vi "mono_camera_array1.vi"(0 "TCP Network Connection in":refnum<k5>, 1 "monoDrive Simulator IP":string, 2 "camera configurations input":T4={"Rear Camera"=path "C:/Users/celit/Documents/GitHub/client/configurations/camera/rear_camera.json", "Left Camera"=path "C:/Users/celit/Documents/GitHub/client/configurations/camera/left_camera.json", "Right Camera"=path "C:/Users/celit/Documents/GitHub/client/configurations/camera/right_camera.json", "Front Camera"=path "C:/Users/celit/Documents/GitHub/client/configurations/camera/front_camera.json", "Following Camera"=path "C:/Users/celit/Documents/GitHub/client/configurations/camera/follow_camera.json"}, 3 "error in (no error)":errorcluster) -> (4 "error out":errorcluster, 5 "camera responses output":T2, 6 "camera dimensions output":T1, 7 "camera connections output":T3, 8 "TCP Network Connection out":refnum<k5>)   [LabVIEW 2018, in "monoDrive.lvlib"]
uses:
  monoDrive.lvlib
panel:
  in  "camera dimensions define":T1
  in  "camera responses define":T2
  in  "camera connections define":T3
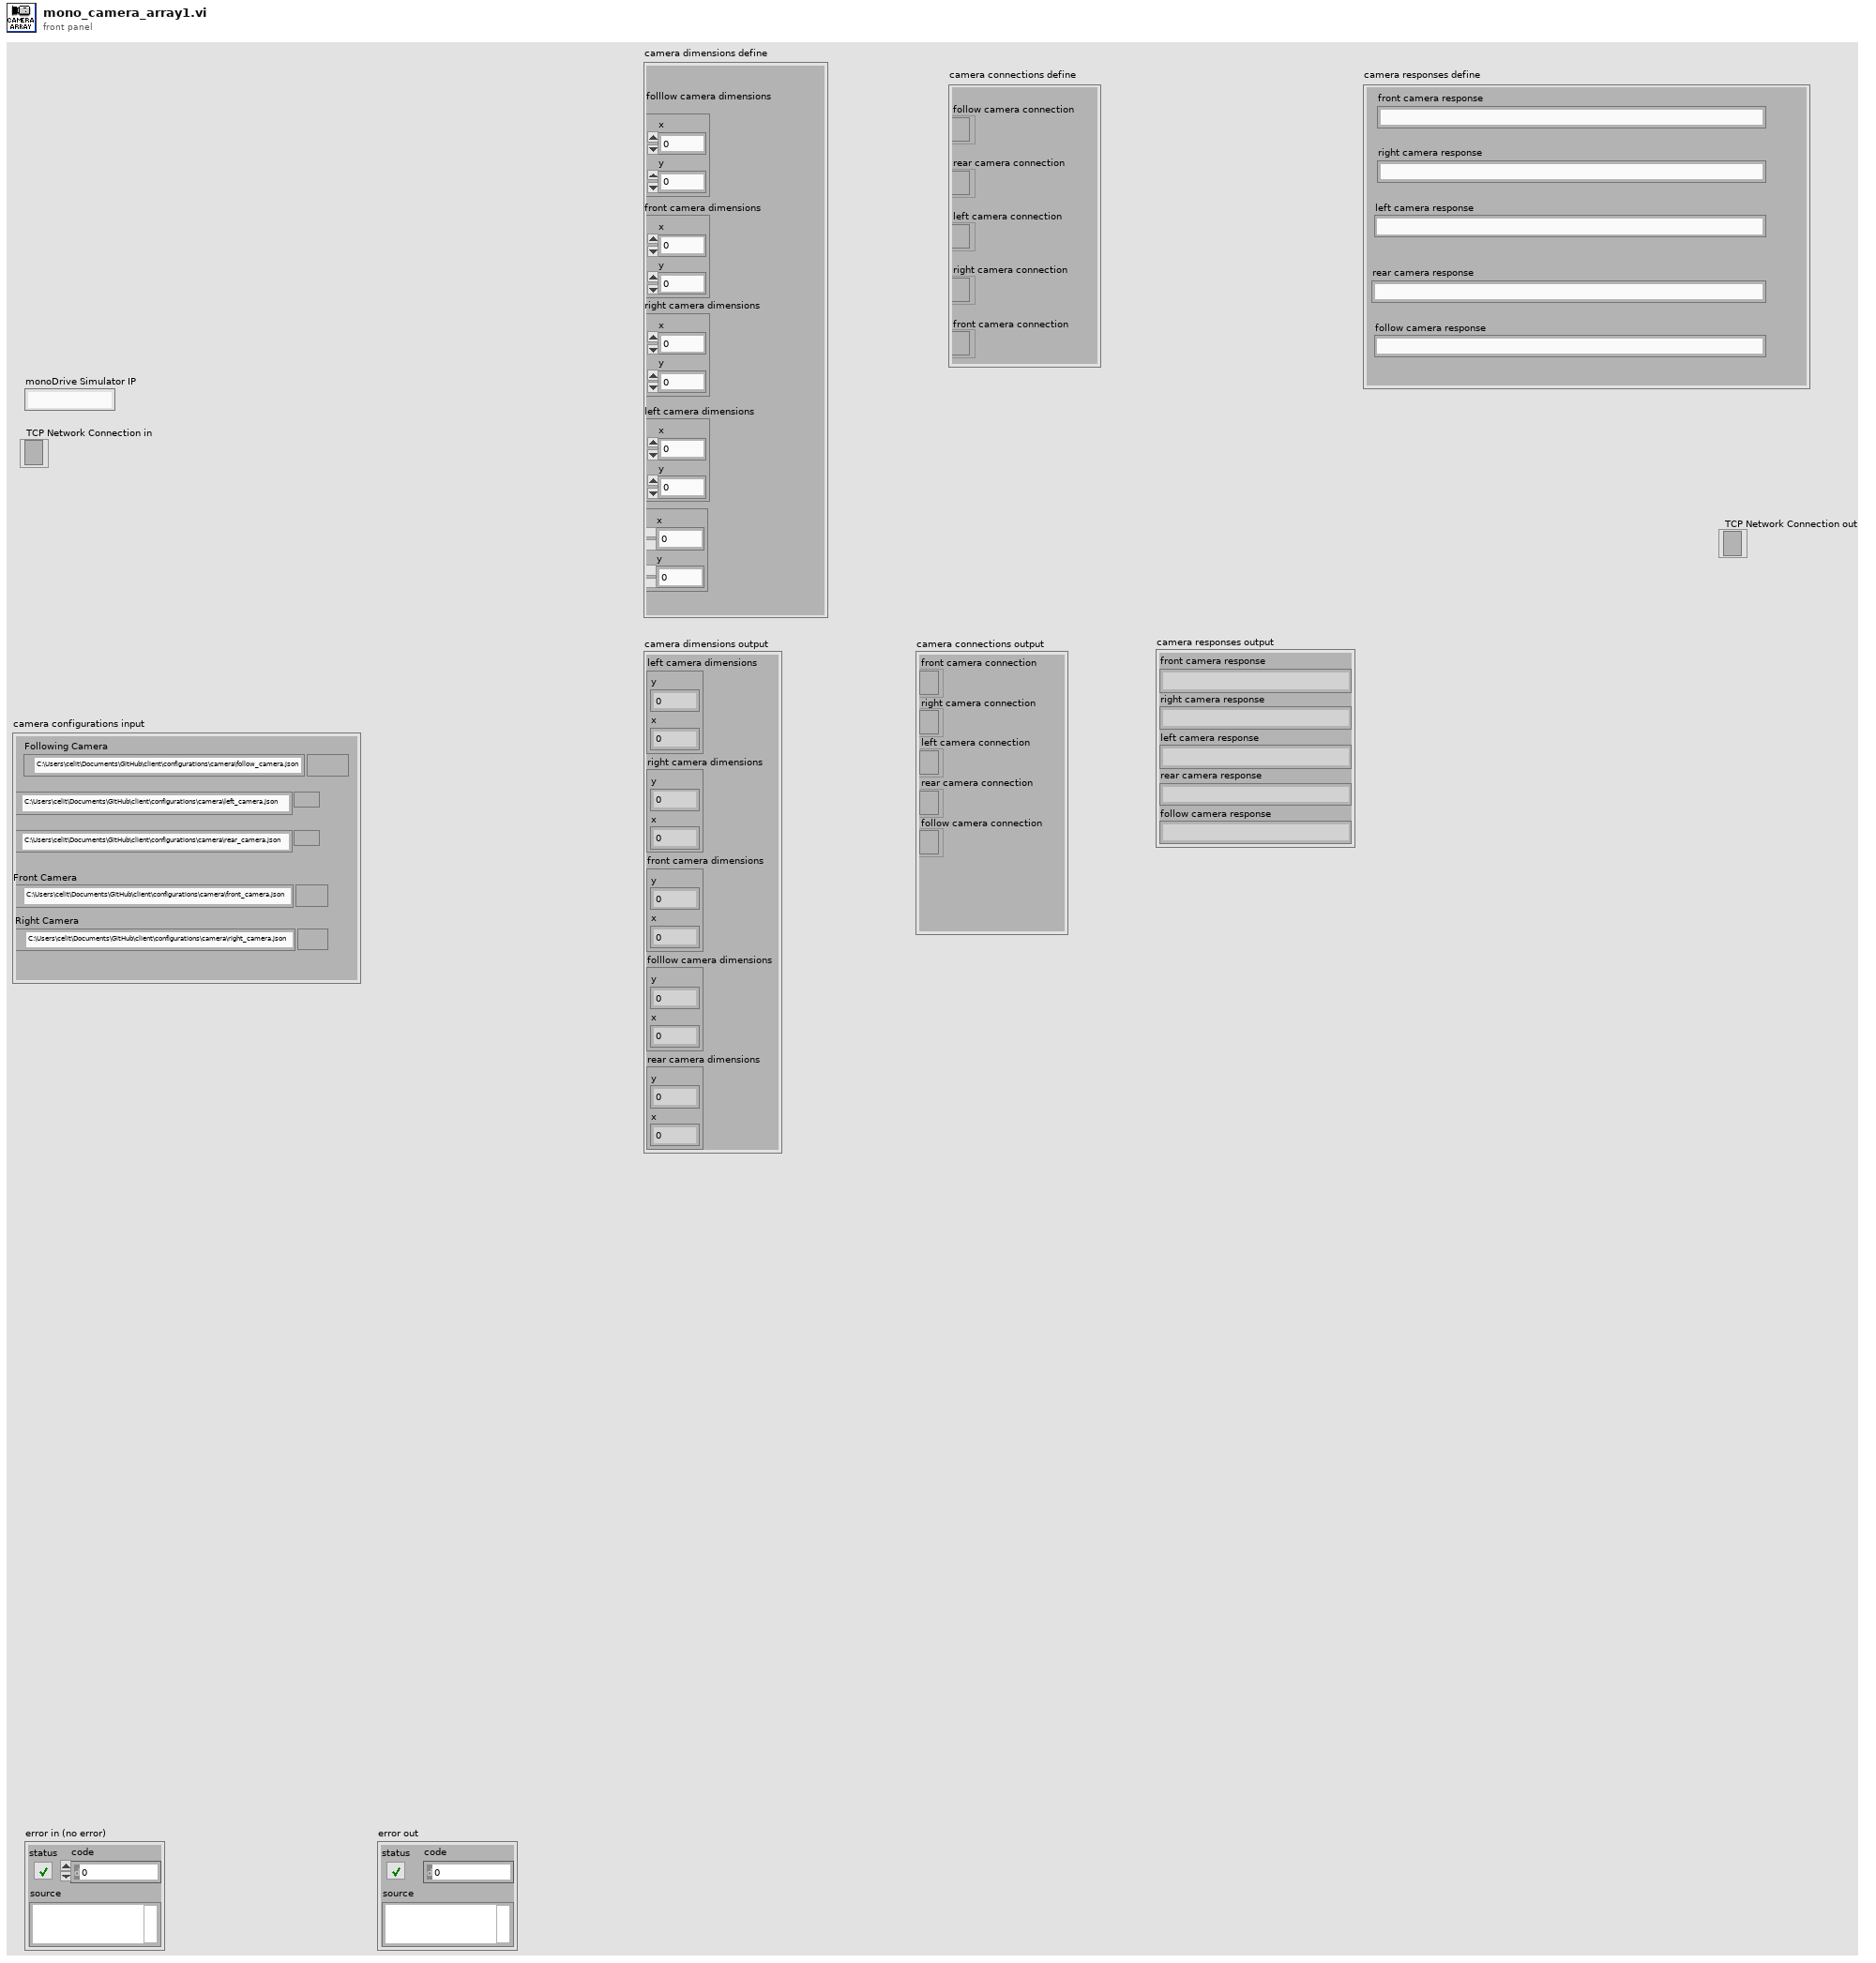
[diagram p1: front panel]
types:
  T1 = cluster{"left camera dimensions":cluster{"y ":i32, "x ":i32}, "right camera dimensions":cluster{"y":i32, "x":i32}, "front camera dimensions":cluster{"y":i32, "x":i32}, "folllow camera dimensions":cluster{"y":i32, "x":i32}, "rear camera dimensions":cluster{"y":i32, "x ":i32}}
  T2 = cluster{"front camera response":string, "right camera response":string, "left camera response":string, "rear camera response":string, "follow camera response":string}
  T3 = cluster{"front camera connection":refnum<k5>, "right camera connection":refnum<k5>, "left camera connection":refnum<k5>, "rear camera connection":refnum<k5>, "follow camera connection":refnum<k5>}
  T4 = cluster{"Rear Camera":path, "Left Camera":path, "Right Camera":path, "Front Camera":path, "Following Camera":path}
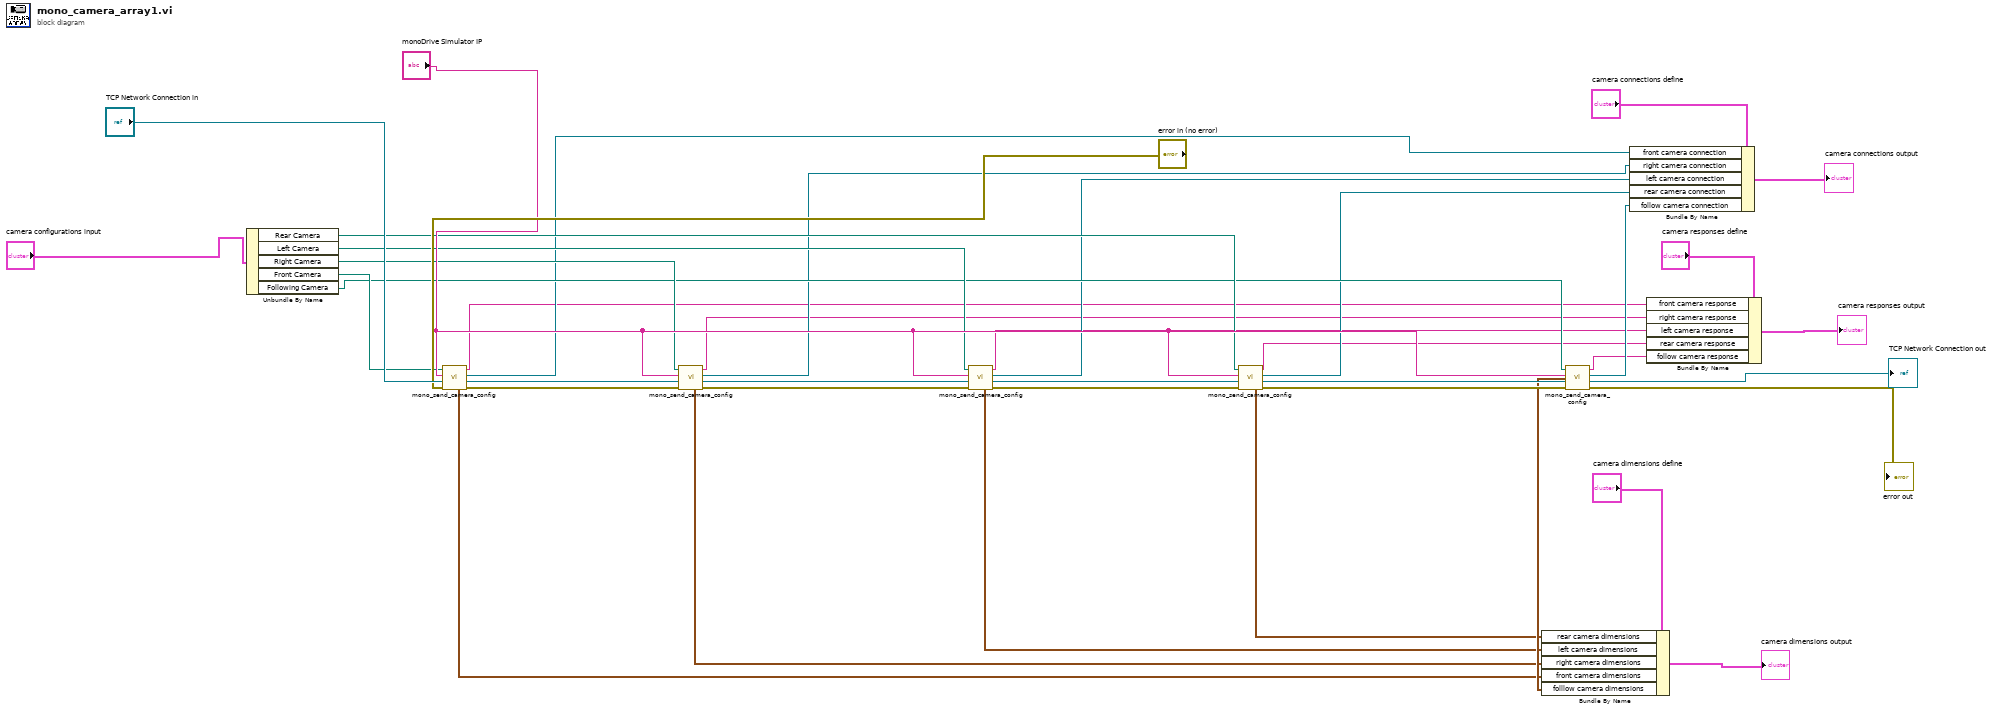
[diagram p0: block diagram]
diagram:
  n1 = Unbundle By Name("camera configurations input") -> ("Rear Camera"=w21:path, "Left Camera"=w20:path, "Right Camera"=w19:path, "Front Camera"=w22:path, "Following Camera"=w18:path)
  n2 = call "mono_send_camera_config.vi"("Camera Configuration Path"=w22, "simulator ip"="monoDrive Simulator IP", "TCP Network Connection in"="TCP Network Connection in", "error in"="error in (no error)") -> ("stream_dimensions"=w27:cluster{"x":i32, "y":i32}, "config response"=w7:string, "sensor connection ID"=w13:refnum<k5>, "TCP Network Connection out"=w33:refnum<k5>, "error out"=w29:errorcluster)
  n3 = call "mono_send_camera_config.vi"("Camera Configuration Path"=w19, "simulator ip"="monoDrive Simulator IP", "TCP Network Connection in"=w33, "error in"=w29) -> ("stream_dimensions"=w26:cluster{"x":i32, "y":i32}, "config response"=w8:string, "sensor connection ID"=w14:refnum<k5>, "TCP Network Connection out"=w34:refnum<k5>, "error out"=w30:errorcluster)
  n4 = call "mono_send_camera_config.vi"("Camera Configuration Path"=w20, "simulator ip"="monoDrive Simulator IP", "TCP Network Connection in"=w34, "error in"=w30) -> ("stream_dimensions"=w25:cluster{"x":i32, "y":i32}, "config response"=w9:string, "sensor connection ID"=w15:refnum<k5>, "TCP Network Connection out"=w35:refnum<k5>, "error out"=w31:errorcluster)
  n5 = call "mono_send_camera_config.vi"("Camera Configuration Path"=w21, "simulator ip"="monoDrive Simulator IP", "TCP Network Connection in"=w35, "error in"=w31) -> ("stream_dimensions"=w24:cluster{"x":i32, "y":i32}, "config response"=w10:string, "sensor connection ID"=w16:refnum<k5>, "TCP Network Connection out"=w36:refnum<k5>, "error out"=w32:errorcluster)
  n6 = call "mono_send_camera_config.vi"("Camera Configuration Path"=w18, "simulator ip"="monoDrive Simulator IP", "TCP Network Connection in"=w36, "error in"=w32) -> ("stream_dimensions"=w28:cluster{"x":i32, "y":i32}, "config response"=w11:string, "sensor connection ID"=w17:refnum<k5>, "TCP Network Connection out"=→"TCP Network Connection out":refnum<k5>, "error out"=→"error out":errorcluster)
  n7 = Bundle By Name(cluster="camera dimensions define", "rear camera dimensions"=w24, "left camera dimensions"=w25, "right camera dimensions"=w26, "front camera dimensions"=w27, "folllow camera dimensions"=w28) -> (→"camera dimensions output":T1)
  n8 = Bundle By Name(cluster="camera connections define", "front camera connection"=w13, "right camera connection"=w14, "left camera connection"=w15, "rear camera connection"=w16, "follow camera connection"=w17) -> (→"camera connections output":T3)
  n9 = Bundle By Name(cluster="camera responses define", "front camera response"=w7, "right camera response"=w8, "left camera response"=w9, "rear camera response"=w10, "follow camera response"=w11) -> (→"camera responses output":T2)
